vi "VideoWriter Set.vi"(8 "error in (no error)":errorcluster, 9 "Value":dbl, 10 "PropId":T1 items=["VIDEOWRITER_PROP_QUALITY"=1, "VIDEOWRITER_PROP_FRAMEBYTES "=2, "VIDEOWRITER_PROP_NSTRIPES "=3, "VIDEOWRITER_PROP_IS_COLOR"=4, "VIDEOWRITER_PROP_DEPTH"=5, "VIDEOWRITER_PROP_HW_ACCELERATION"=6, "VIDEOWRITER_PROP_HW_DEVICE"=7, "VIDEOWRITER_PROP_HW_ACCELERATION_USE_OPENCL"=8, "VIDEOWRITER_PROP_RAW_VIDEO"=9, "VIDEOWRITER_PROP_KEY_INTERVAL"=10, "VIDEOWRITER_PROP_KEY_FLAG "=11, "IDEOWRITER_PROP_PTS"=12, "VIDEOWRITER_PROP_DTS_DELAY"=13], 11 "VideoWriter in":refnum<class "VideoWriter.lvclass">) -> (0 "error out":errorcluster, 2 "Success":bool, 3 "VideoWriter out":refnum<class "VideoWriter.lvclass">)   [LabVIEW 2020, in "OpenLvVision_OpenCv.lvlib" / "VideoWriter.lvclass"]
doc: "Sets a property in the VideoWriter."
uses:
  VideoWriter.lvclass
  OpenLvVision_OpenCv.lvlib
  _LvHelpers/EdvrObject/EdvrObject.lvclass
  C:/Users/lukas/Downloads/OpenLvVision_OpenCv/SourceCode/LabView/OpenLvVision_OpenCv/_LvHelpers/EdvrObject/EdvrObject.lvclass
  Dlls/OlvOpenCvWrapper.dll
  TypeDef/VideoWriterProperties.ctl
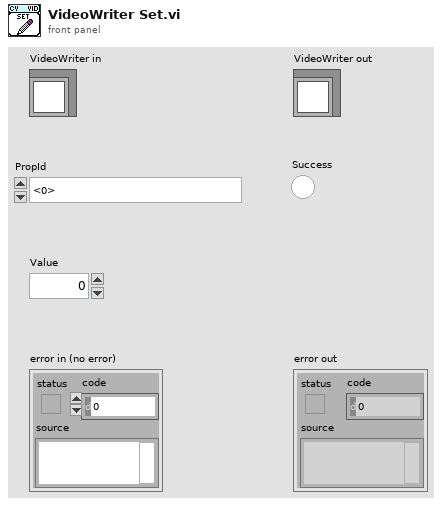
[diagram p1: front panel]
types:
  T1 = typedef "OpenLvVision_OpenCv.lvlib/VideoWriterProperties.ctl" = i32
  T2 = typedef "OpenLvVision_OpenCv.lvlib/EdvrObject.lvclass/Edvr.ctl" = refnum<data-value>
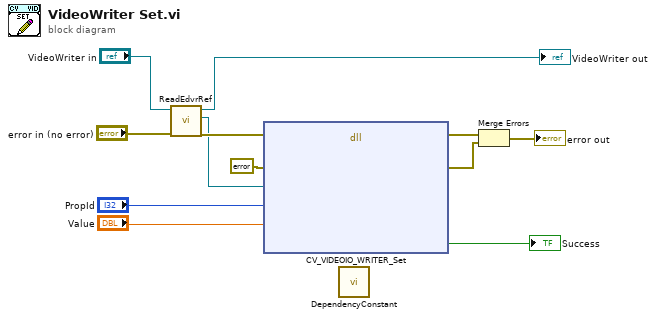
[diagram p0: block diagram]
diagram:
  n1 = call "ReadEdvrRef.vi"("error in (no error)"="error in (no error)", "EdvrObject in"="VideoWriter in") -> ("error out"=w11:errorcluster, "Edvr"=w10:T2, "EdvrObject out"=→"VideoWriter out":refnum<class "VideoWriter.lvclass">)  [unwired: 7 in]
  n2 = dll-call lib="C:/Users/lukas/Downloads/OpenLvVision_OpenCv/SourceCode/LabView/OpenLvVision_OpenCv/Dlls/OlvOpenCvWrapper.dll" fn="CV_VIDEOIO_WRITER_Set"(error in=w11, "Error"=errorcluster {"status"=FALSE, "code"=0, "source"=""} ("error out"), "edvrRef"=w10, "propId"="PropId", "value"="Value") -> (error out=w9:errorcluster, "Error"=w6:errorcluster, "Success"=→"Success":bool)  [unwired: 7 in, 1 out]
  n3 = call "DependencyConstant.vi"() -> ()  [unwired: 12 in]
  n4 = Merge Errors(w9, w6) -> (→"error out":errorcluster)
